vi "get_username.vi"(8 "error in (no error)":errorcluster, 9 "string in":string) -> (0 "error out":errorcluster, 1 "edited string out":string)   [LabVIEW 2010, in "ErrorController.lvclass"]
uses:
  ErrorController.lvclass
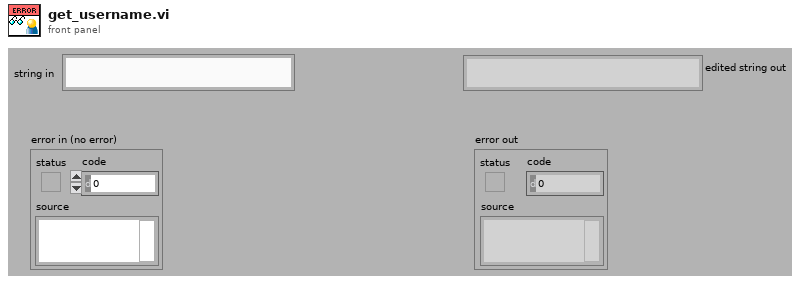
[diagram p1: front panel]
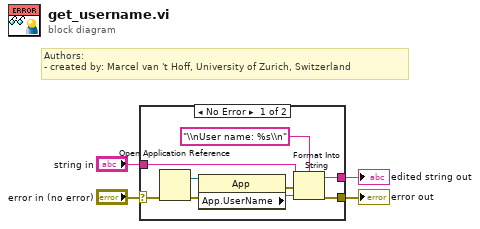
[diagram p0: block diagram]
diagram:
  # "Authors: \n- created by: Marcel van 't Hoff, University of Zurich, Switzerland"
  n1 = case shown="No Error" "error in (no error)" {
    selector: "error in (no error)" -> [w5 w14]
    tunnel: [w6 w14] -> w3
    tunnel: "string in" -> [w11 _]
    tunnel: [w7 _] -> w1
    frame No Error {
      n2 = Open Application Reference(8:w5) -> (0:w12:errorcluster, 3:w13:refnum<vi>)  [unwired: 3 in]
      n3 = property class="App"(reference=w13, error in=w12) -> (error out=w9:errorcluster, "App.UserName"=w8:string)  [unwired: 1 out]
      n4 = Format Into String(format string="\\nUser name: %s\\n", initial string=w11, error in=w9, w8) -> (resulting string=w7:string, error out=w6:errorcluster)
    }
    frame Error {
    }
  }
  "error out" <- w3
  "edited string out" <- w1
